vi "MiniWheel Control Code Comprehensive.vi"() -> ()   [LabVIEW 2016]
uses:
  <userlib>/dynamixel32bit/dynamixel.lvlib
panel:
  out "Wheel Motor Position V. Time 3":i32(graph)
  in  "# of Steps per Gait Cycle":dbl
  in  "Angle Increment per Step":dbl
  in  "Theta Naught":dbl
  in  "Step Delay (Seconds)":dbl
  in  "Baud Rate":i32=1
  in  "Com Port":i32=3
  in  "Wheel Speed":u16=512 max=1023 step=1
  in  "Wheel Dynamixel ID":i32=1
  out "Rotator Motor Position V. Time":i32(graph)
  in  "Rotator Dynamixel ID":i32=1
  in  "stop":bool
  out "Present Position":u16(slide) max=1023 scale=0.0..1023.0
  # "Instructions:\n1) Enter Initialization Parameters\n2) Enter Parameters\n3) Click START Motors button\n4) Change values as desired during run"
  # "Motor Feedback"
  # "Initialization"
  # "ID 12"
  # "COM 16"
  # "Baud 1"
  # "ID 6"
  # "Parameters"
  # "Common Values by Gait:\n     Wave Gait:\n          Step Delay:\n          Theta Naught:\n          Angle Increment:\n          # of Steps/cycle:\n     RP Gait:\n          Step Delay:\n          Theta Naught:\n          Angle Increment:\n          # of Steps/cycle:\n     Rear Rotator Pedaling Gait:\n          Step Delay:\n          Theta Naught:\n          Angle Increment:\n          # of Steps/cycle:"
  # "Example: 256 + 12(21.333) = 512"
  # "Note: Position graphs will NOT operate during gait operation"
  # "256"
  # "+"
  # "21.333"
  # "x"
  # "12"
  # "= 512"
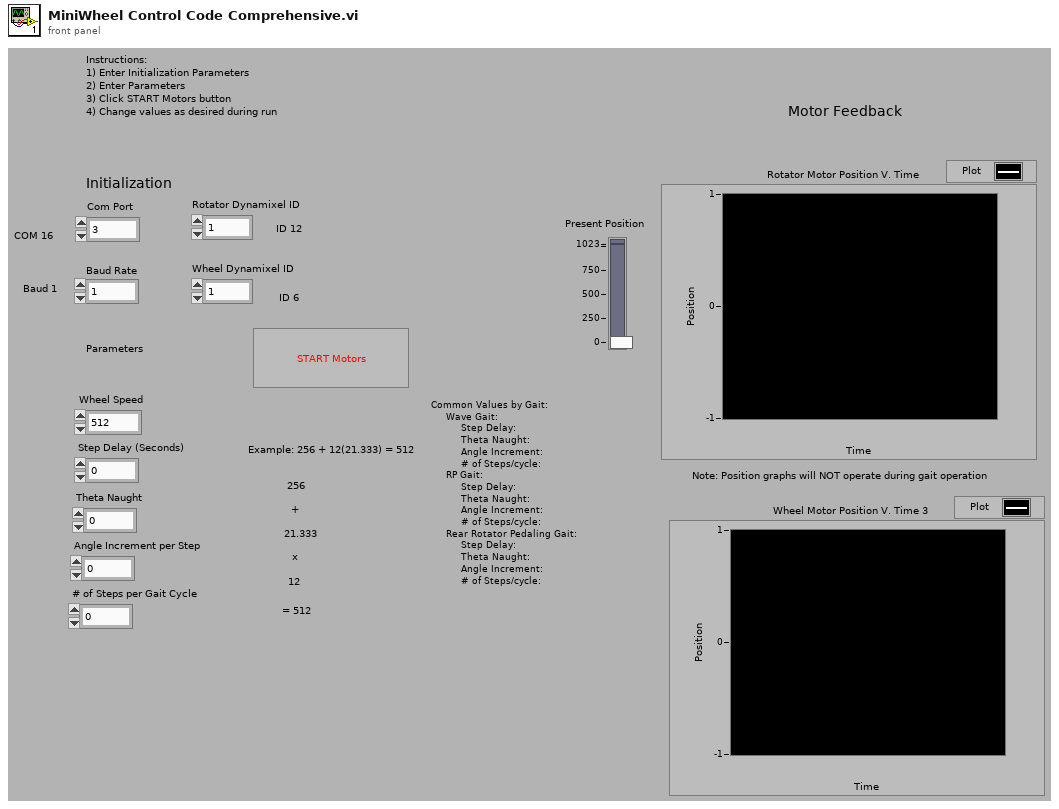
[diagram p1: front panel]
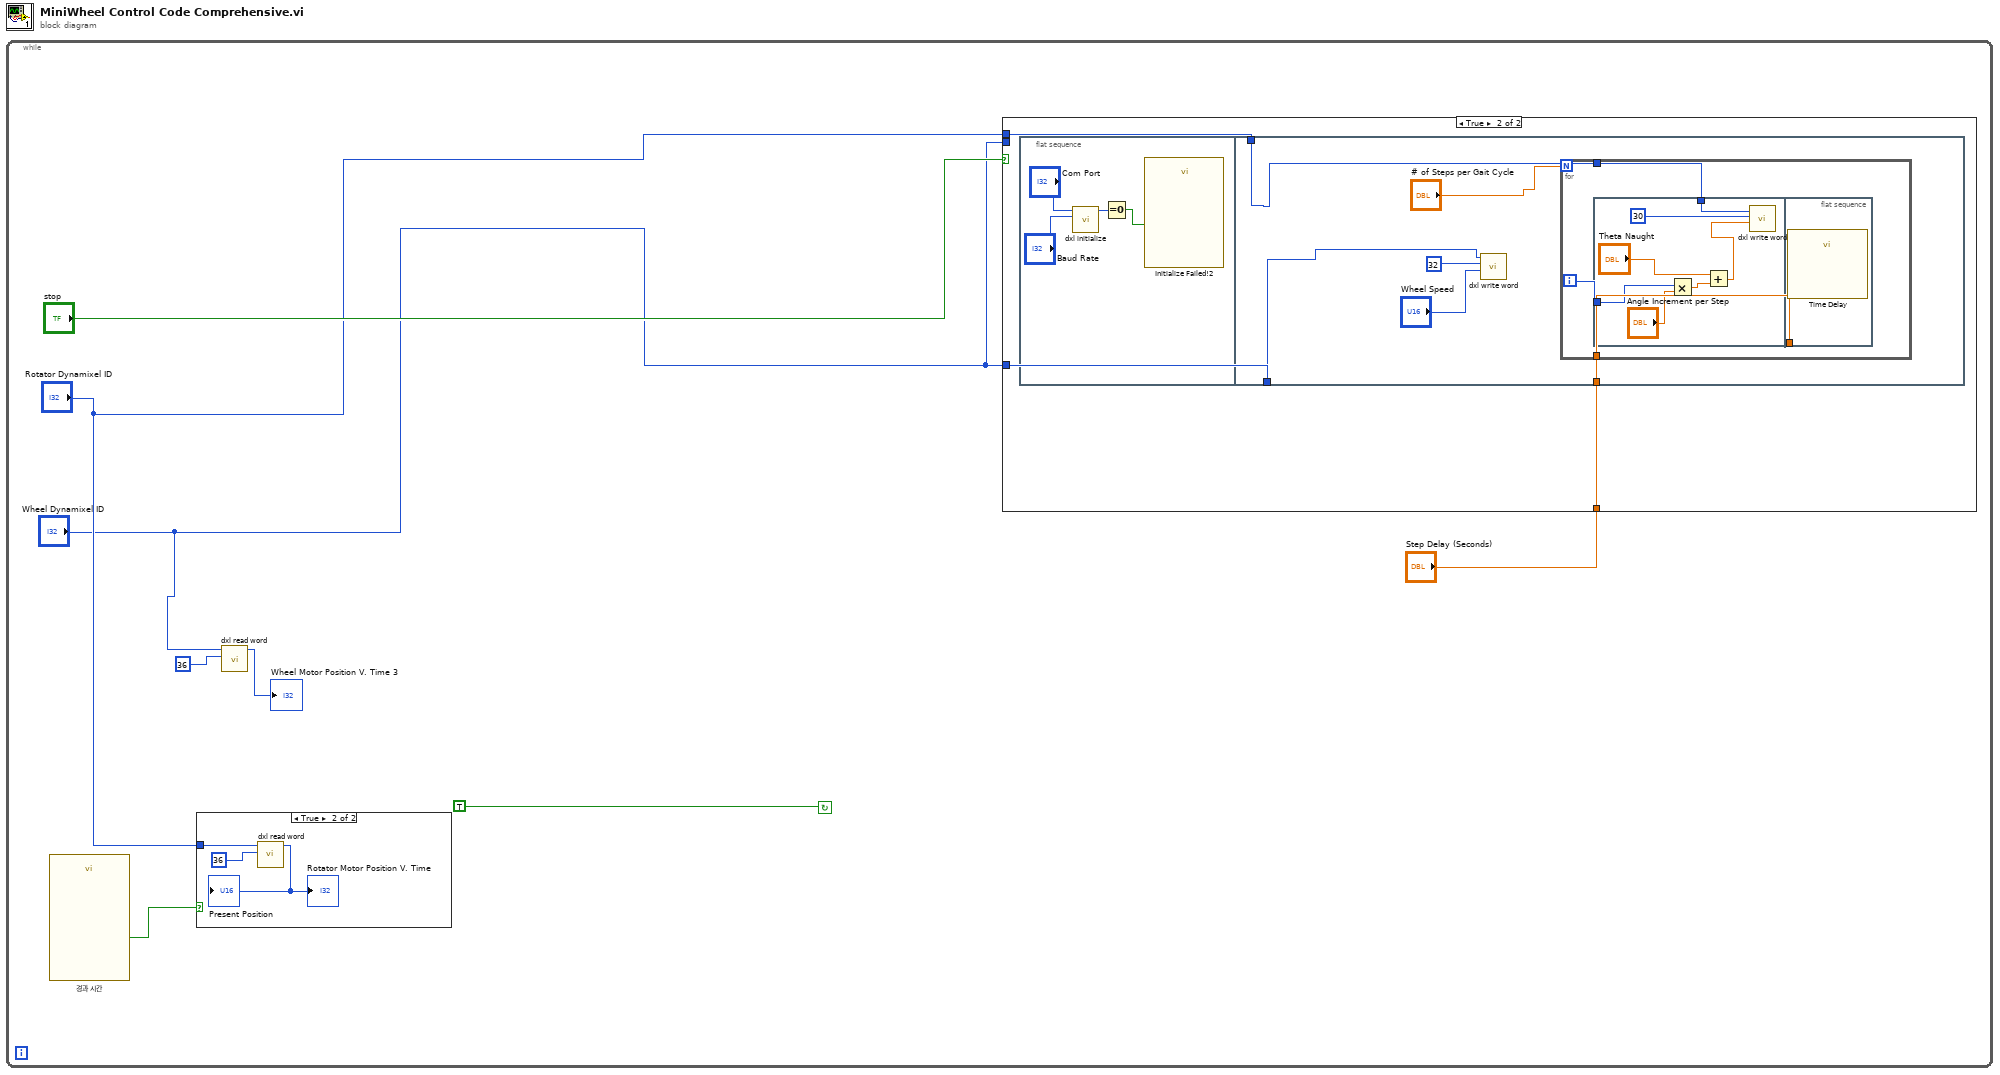
[diagram p0: block diagram]
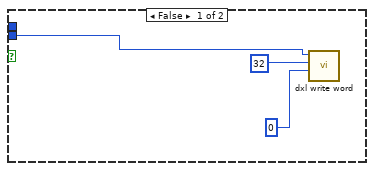
[diagram p2: hidden frame]
diagram:
  n1 = while {
    stop <- TRUE continue-if-true
    n2 = call "경과 시간"() -> ("Time has Elapsed"=w7:bool)  [unwired: 12 in, 7 out]
    n3 = case shown="True" w7 {
      tunnel: "Rotator Dynamixel ID" -> [_ w38]
      frame False {
      }
      frame True {
        n4 = call <userlib>:"dxl read word.vi"("address"=36, "id"=w38) -> ("function return"=→"Present Position" →"Rotator Motor Position V. Time":i32)  [unwired: 9 in]
      }
    }
    n5 = call <userlib>:"dxl read word.vi"("address"=36, "id"="Wheel Dynamixel ID") -> ("function return"=→"Wheel Motor Position V. Time 3":i32)  [unwired: 9 in]
    n6 = case shown="True" "stop" {
      tunnel: "Wheel Dynamixel ID" -> [w10 _]
      tunnel: "Rotator Dynamixel ID" -> [_ w14]
      tunnel: "Wheel Dynamixel ID" -> [_ w13]
      tunnel: "Step Delay (Seconds)" -> [_ w12]
      frame False {
        n7 = call <userlib>:"dxl write word.vi"("value"=0, "address"=32, "id"=w10) -> ()  [unwired: 9 in]
      }
      frame True {
        n8 = flat-sequence {
          tunnel: w14 -> [w22]
          tunnel: w13 -> [w21]
          tunnel: w12 -> [w20]
          frame #0 {
            n9 = call <userlib>:"dxl initialize.vi"("baudnum"="Baud Rate", "devIndex"="Com Port") -> ("function return"=w17:i32)  [unwired: 9 in]
            n10 = Equal To 0?(x=w17) -> (x = 0?=w18:bool)
            n11 = call "Initialize Failed!2"("Enable"=w18) -> ()  [unwired: 9 in, 2 out]
          }
          frame #1 {
            n12 = call <userlib>:"dxl write word.vi"("value"="Wheel Speed", "address"=32, "id"=w21) -> ()  [unwired: 9 in]
            n13 = for {
              N: "# of Steps per Gait Cycle" -> [_]
              tunnel: w22 -> [w27]
              tunnel: w20 -> [w25]
              i -> [w26]
              n14 = flat-sequence {
                tunnel: w27 -> [w33]
                tunnel: w26 -> [w32]
                tunnel: w25 -> [w35]
                frame #0 {
                  n15 = Multiply(x=w32, y="Angle Increment per Step") -> (x*y=w31:dbl)
                  n16 = Add(x="Theta Naught", y=w31) -> (x+y=w30:dbl)
                  n17 = call <userlib>:"dxl write word.vi"("value"=w30, "address"=30, "id"=w33) -> ()  [unwired: 9 in]
                }
                frame #1 {
                  n18 = call "Time Delay"("Delay Time (s)"=w35) -> ()  [unwired: 10 in, 1 out]
                }
              }
            }
          }
        }
      }
    }
  }
